vi "Get SubpanelVI Info.vi"(8 "error in (no error)":errorcluster, 11 "Configuration in":refnum<class "UserPwd DB Configuration.lvclass">) -> (0 "error out":errorcluster, 1 "Subpanel VI data":T1, 2 "Category string":string, 3 "Configuration out":refnum<class "UserPwd DB Configuration.lvclass">)   [LabVIEW 2016, in "UserPwd DB.lvlib" / "UserPwd DB Configuration.lvclass"]
uses:
  <userlib>/Common Components/UserPwd DB/UserPwd DB Config/UserPwd DB Configuration.lvclass
  <userlib>/Configuration Dialog Actor/Methods/Data Retrieved by Lookup Table.ctl
  <userlib>/Configuration Dialog Actor/Configuration.lvclass
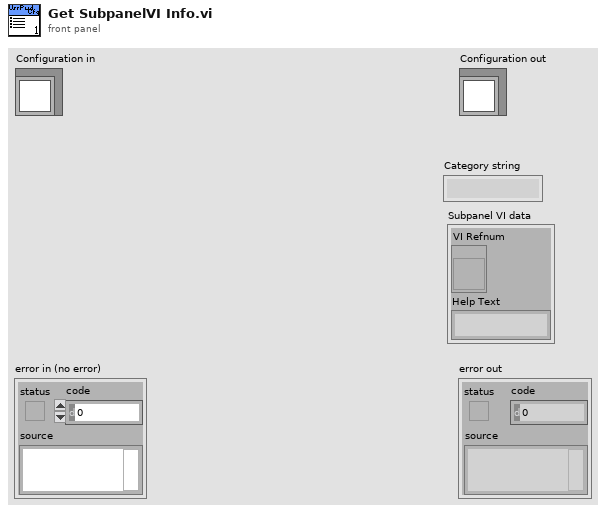
[diagram p1: front panel]
types:
  T1 = typedef "Configuration.lvlib/Configuration.lvclass/Data Retrieved by Lookup Table.ctl" = cluster{"VI Refnum":refnum<vi>, "Help Text":string}
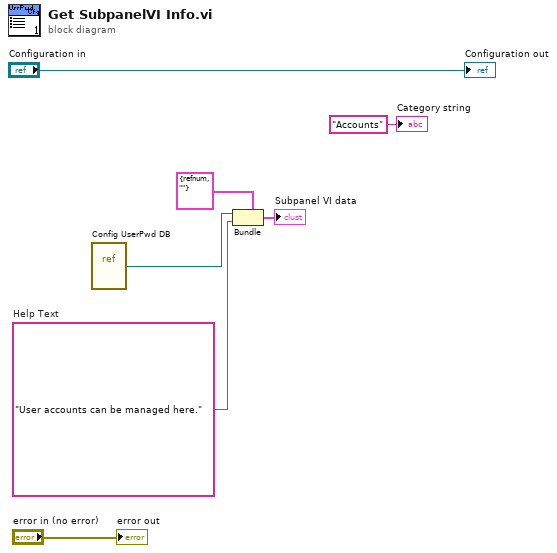
[diagram p0: block diagram]
diagram:
  w3 = "User accounts can be managed here."  # Help Text
  n1 = vi-ref <userlib>:"Config UserPwd DB.vi"() -> (w4:refnum<vi>)
  n2 = Bundle(cluster=T1 {"VI Refnum"=refnum, "Help Text"=""} ("output cluster"), "VI Refnum"=w4, "Help Text"=w3) -> (→"Subpanel VI data":T1)
  "error out" <- "error in (no error)"
  "Configuration out" <- "Configuration in"
  "Category string" <- "Accounts" ("Category string")
